vi "Draw Single Note.vi"(5 "Clef":T1, 6 "Line Spacing":i16=30, 7 "Note Number":i16=2, 8 "Start y":i16=215, 9 "Start x":i16=80, 10 "Picture Path":path=path "C:/Users/jag2k2/Desktop/Flashcards", 11 "Picture In":picture) -> (3 "Picture Out":picture)   [LabVIEW 2014]
uses:
  Type Defs/Clef.ctl
panel:
  in  "Reg Line Note Offset 2":i16=-15
  in  "Invt Line Note Offset 2":i16=15
  in  "Reg Line Note Offset":i16=-15
  in  "Invt Line Note Offset":i16=15
  in  "Invt Offset 2":i16=75
  in  "Invt Line Offset 2":i16=15
  in  "Reg Line Offset 2":i16=105
  in  "Reg Offset 2":i16=-15
  in  "Invt Offset":i16=15
  in  "Invt Line Offset":i16=15
  in  "Reg Line Offset":i16=105
  in  "Reg Offset":i16=-75
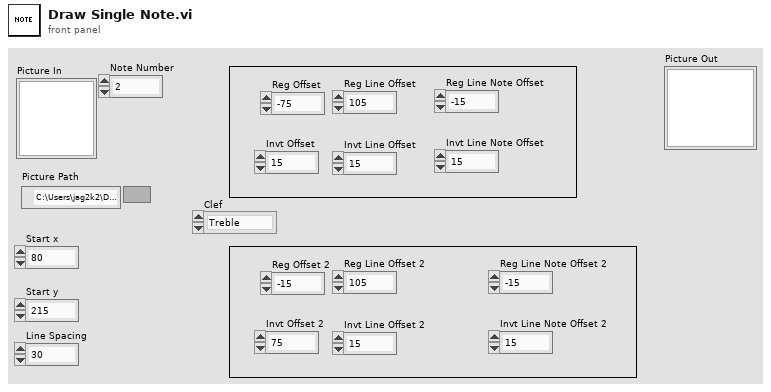
[diagram p1: front panel]
types:
  T1 = typedef "Clef.ctl" = enum16{"Treble", "Bass"}
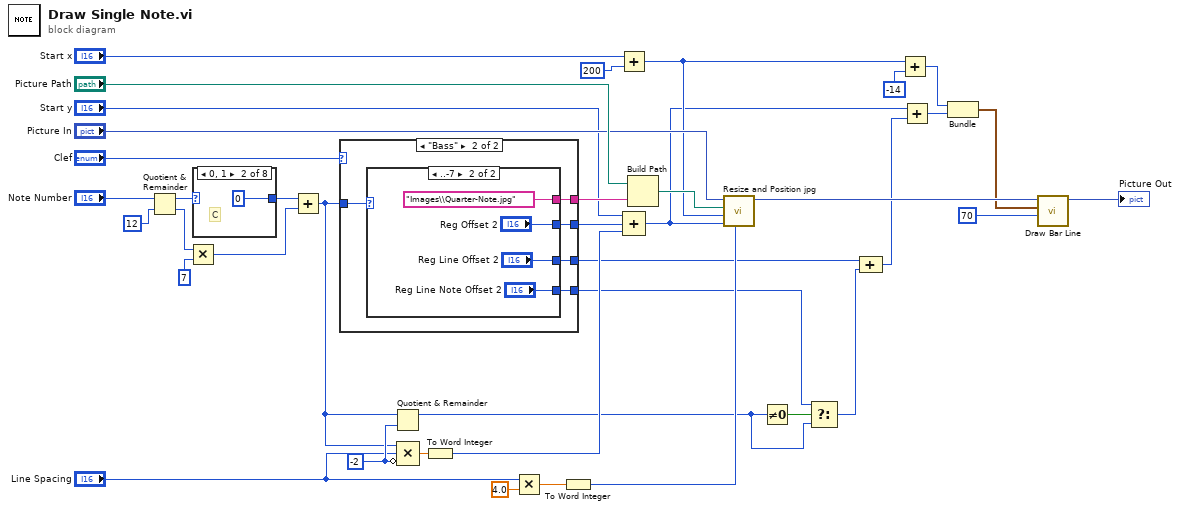
[diagram p0: block diagram]
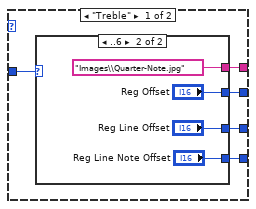
[diagram p2: hidden frame]
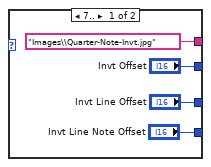
[diagram p3: hidden frame]
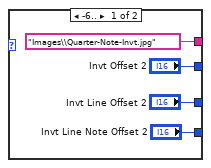
[diagram p4: hidden frame]
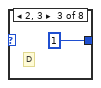
[diagram p6: hidden frame]
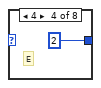
[diagram p7: hidden frame]
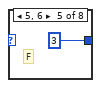
[diagram p8: hidden frame]
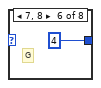
[diagram p9: hidden frame]
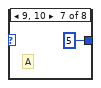
[diagram p10: hidden frame]
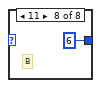
[diagram p11: hidden frame]
diagram:
  w25 = i16 -2 ("value")
  n1 = Quotient & Remainder(x="Note Number", y=i16 12) -> (x-y*floor(x/y)=w16:i16, floor(x/y)=w17:i16)
  n2 = Multiply(x=w17, y=i16 7) -> (x*y=w18:i16)
  n3 = case shown="0, 1" w16 {
    tunnel: [_ i16 0 ("Note Number") i16 1 ("Note Number") i16 2 ("Note Number") i16 3 ("Note Number") i16 4 ("Note Number") i16 5 ("Note Number") i16 6 ("Note Number")] -> w19
    frame Default {
    }
    frame 0, 1 {
      # "C"
    }
    frame 2, 3 {
      # "D"
    }
    frame 4 {
      # "E"
    }
    frame 5, 6 {
      # "F"
    }
    frame 7, 8 {
      # "G"
    }
    frame 9, 10 {
      # "A"
    }
    frame 11 {
      # "B"
    }
  }
  n4 = Add(x=w19, y=w18) -> (x+y=w3:i16)
  n5 = case shown="\"Bass\"" "Clef" {
    tunnel: [w51 w64] -> w37
    tunnel: [w50 w63] -> w29
    tunnel: w3 -> [w49 w62]
    tunnel: [w48 w61] -> w8
    tunnel: [w47 w60] -> w1
    frame "Treble" {
      n6 = case shown="..6" w49 {
        tunnel: ["Images\\Quarter-Note-Invt.jpg" ("name or relative path") "Images\\Quarter-Note.jpg" ("name or relative path")] -> w51
        tunnel: ["Invt Offset" "Reg Offset"] -> w50
        tunnel: ["Invt Line Offset" "Reg Line Offset"] -> w48
        tunnel: ["Invt Line Note Offset" "Reg Line Note Offset"] -> w47
        frame 7.. {
        }
        frame ..6 {
        }
      }
    }
    frame "Bass" {
      n7 = case shown="..-7" w62 {
        tunnel: ["Images\\Quarter-Note-Invt.jpg" ("name or relative path") "Images\\Quarter-Note.jpg" ("name or relative path")] -> w64
        tunnel: ["Invt Offset 2" "Reg Offset 2"] -> w63
        tunnel: ["Invt Line Offset 2" "Reg Line Offset 2"] -> w61
        tunnel: ["Invt Line Note Offset 2" "Reg Line Note Offset 2"] -> w60
        frame -6.. {
        }
        frame ..-7 {
        }
      }
    }
  }
  n8 = Quotient & Remainder(x=w3, y=w25) -> (x-y*floor(x/y)=w2:i16)  [unwired: 1 out]
  n9 = Compound Arithmetic op=MULTIPLY(w3, "Line Spacing", invert w25) -> (w31:dbl)
  n10 = To Word Integer(number=w31) -> (16bit integer=w30:i16)
  n11 = Multiply(x="Line Spacing", y=4.0 ("y 3")) -> (x*y=w35:dbl)
  n12 = To Word Integer(number=w35) -> (16bit integer=w34:i16)
  n13 = Add(x="Start x", y=i16 200) -> (x+y=w24:i16)
  n14 = Compound Arithmetic op=ADD("Start y", w29, w30) -> (w22:i16)
  n15 = Build Path(base path="Picture Path", name or relative path=w37) -> (appended path=w39:path)
  n16 = call "Resize and Position jpg.vi"("New Height"=w34, "Pos y"=w22, "Pos x"=w24, "appended path"=w39, "Picture In"="Picture In") -> ("Picture Out"=w27:picture)  [unwired: 6 in]
  n17 = Not Equal To 0?(x=w2) -> (x != 0?=w10:bool)
  n18 = Select(t=w1, s=w10, f=w2) -> (s? t:f=w7:i16)
  n19 = Compound Arithmetic op=ADD(w8, w7) -> (w6:i16)
  n20 = Add(x=w24, y=i16 -14 ("x")) -> (x+y=w12:i16)
  n21 = Add(x=w22, y=w6) -> (x+y=w13:i16)
  n22 = Bundle(w12, w13) -> (w14:cluster{i16, i16})  [unwired: 1 in]
  n23 = call "Draw Bar Line.vi"("Line Length"=i16 70, "end point"=w14, "picture in"=w27) -> ("picture out"=→"Picture Out":picture)  [unwired: 8 in]
